vi "Plate Tank 1.vi"() -> ()   [LabVIEW 2019]
uses:
  <vilib>/NI/Current Value Table/Type Defs/Single Tag.ctl
  <vilib>/NI/Current Value Table/Type Defs/Data Types.ctl
  <vilib>/Utility/sysdir.llb/System Directory Type.ctl
  <vilib>/NI/STM/TCP/Read Meta Data (TCP Ref).vi
  <vilib>/NI/STM/TCP/Get Connection Reference (TCP).vi
  <vilib>/NI/AMC/Read Termination Message.vi
  <vilib>/NI/AMC/Create Single Message.vi
  <vilib>/NI/AMC/Update Message Routing Info.vi
  <vilib>/NI/STM/TCP/Read Meta Data (TCP Clst).vi
  <vilib>/NI/AMC/Send Message.vi
  <vilib>/NI/AMC/Globals.vi
  <userlib>/_OpenG.lib/comparison/comparison.llb/I32 Changed__ogtk.vi
  <vilib>/NI/STM/TCP/Write Message (TCP).vi
  <vilib>/NI/AMC/AMC.lvlib
  <vilib>/NI/STM/NI STM.lvlib
  <vilib>/NI/Current Value Table/Current Value Table.lvlib
panel:
  in  "EZ Recipe Button":bool
  out "Loaded Recipe":string
  in  "Load A Recipe":bool
  in  "Save This Recipe":bool
  out "Right Time":dbl format="%.1f"
  out "Left Time":dbl format="%.1f"
  out "Total Amp*min R":dbl format="%.1f"
  out "Total Amp*min L":dbl format="%.1f"
  in  "MO":string
  in  "Reverse Current Multiplier":dbl=3.0 min=0.1 max=100.0 step=0.01 format="%.2g"
  in  "Rectifer Settings":i32(listbox)
  in  "BasT1_P Last Hr":bool
  in  "BasT1_Level Last Hr":bool
  out "Boolean 5":bool
  out "SumpBottom":bool
  out "Process 1 Supply":bool
  out "Sump Return":bool
  out "Boolean 2":bool
  out "SG":dbl format="%.3g"
  out "Return to sump 4":bool
  in  "Rectifer Data":enum32{"Standard", "Eng"}(tab)
  out "Current Step":i32
  out "Left Anode Actual Current":dbl(knob) scale=0.0..150.0
  out "Right Anode Actual Current":dbl(knob) scale=0.0..150.0
  out "Left Anode Amp-min":dbl(slide) scale=0.0..254.0
  out "Right Anode Amp-min":dbl(slide) scale=0.0..135.0
  out "Output Voltage":cluster{dbl, dbl}(graph)
  in  "Tab Control 2":enum32{"Standard", "ENG"}(tab)
  out "Supply Flow":dbl(knob) scale=0.0..65.0
  out "Plating Cell Liquid Level":dbl(slide) scale=0.0..75.0
  out "Cell Temperature":dbl(slide) scale=0.0..60.0
  in  "Cell T Last Hr":bool
  out "Suck Pump":bool
  out "Suck Pump Flow":dbl format="%#_4g"
  out "SuckPipe":bool
  out "SuckPipe 3":bool
  out "Drain Tee Top":bool
  out "Return to sump 2":bool
  out "Return to sump 3":bool
  out "Flow Controller":dbl(knob) scale=0.0..100.0
  in  "Tab Control":enum32{"Main Pump", "Suck Pump"}(tab)
  out "Amps":dbl format="%#.2g"
  out "Volts":dbl format="%#.1f"
  out "VFD T":dbl format="%#.2g"
  out "RPM":dbl format="%#.0f"
  out "Fault Code":dbl format="%#.2g"
  out "Freq":dbl format="%#.2g"
  out "SP1 Amps":dbl caption="Amps" format="%#.2g"
  out "SP1 Volts":dbl caption="Volts" format="%#.1g"
  out "SP1 RPM":dbl caption="RPM" format="%#.2g"
  out "SP1 VFD T":dbl caption="VFD T" format="%#.2g"
  out "SP1 Fault Code":dbl caption="Fault Code" format="%#.2g"
  out "SP1 Freq":dbl caption="Freq" format="%#.2g"
  out "Flow 1":dbl format="%#_4g"
  out "Flow 2":dbl format="%#_4g"
  out "Flow 3":dbl format="%#_4g"
  out "Flow 4":dbl format="%#_4g"
  out "Return to sump":bool
  out "E Stop":bool
  out "Run Enabled?":bool
  in  "Full Drain Plating Cell":bool
  out "Rack Motion":bool
  out "Right Eductor Motion":bool
  out "Left Eductor Motion":bool
  out "Right Output On":bool
  in  "Enable Rack Motion":bool
  in  "Rack RPM":dbl(knob)=1.0 min=1.0 max=11.0 step=0.03 scale=0.0..11.0
  out "Left Output On":bool
  in  "Start Cycle":bool
  in  "Cancel Cycle":bool
  out "SuckPipe 2":bool
  out "Main Pump":bool
  in  "Enable Eductor Motion":bool
  in  "Eductor RPM":dbl(knob)=1.0 min=1.0 max=11.0 step=0.05 scale=0.0..11.0
  in  "Supply Pressure (kPa)":dbl(knob)=50.0 min=50.0 max=200.0 step=5.0 scale=50.0..200.0
  in  "Total Inflow (L/min)":dbl(knob)=40.0 min=25.0 max=50.0 step=0.5 scale=25.0..50.0
  in  "Suck Pump fraction of inflow":dbl(knob)=5.0 min=5.0 max=90.0 step=1.0 scale=0.0..90.0
  out "Sump Level":dbl(slide) scale=0.0..1000.0
  out "Supply Pressure":dbl(knob) scale=0.0..200.0
  in  "Enable Suck Pump":bool
  in  "Enable Plating Cell":bool
  in  "Machine":bool
  in  "Basement 4":bool
  in  "Dryer":bool
  in  "Rinse 4":bool
  in  "Rinse 3":bool
  in  "Rinse 2":bool
  in  "Basement 3":bool
  in  "Basement 2":bool
  in  "Basement 1":bool
  in  "Plater 6":bool
  in  "Plater 5":bool
  in  "Plater 4":bool
  in  "Plater 3":bool
  in  "Plater 2":bool
  in  "Plater 1":bool
  in  "Predip":bool
  in  "Rinse 1":bool
  in  "Cleaner":bool
  in  "Etch":bool
  out "status":string
  out "Boolean 4":bool
  # "Module Selection"
  # "Rectifier Settings"
  # "Fluid Flow Control"
  # "(mins)"
  # "Rectifier Control"
  # "Rectifier Output"
  # "Motion starts when rectifiers cycle"
  # "Note: RPM settings shared with tank 2"
  # "kPa"
  # "@"
  # "Output"
  # "cm"
  # "°C"
  # "L/min"
  # "cm"
  # "L/min"
  # "L/min"
  # "L/min"
  # "L/min"
  # "L/min"
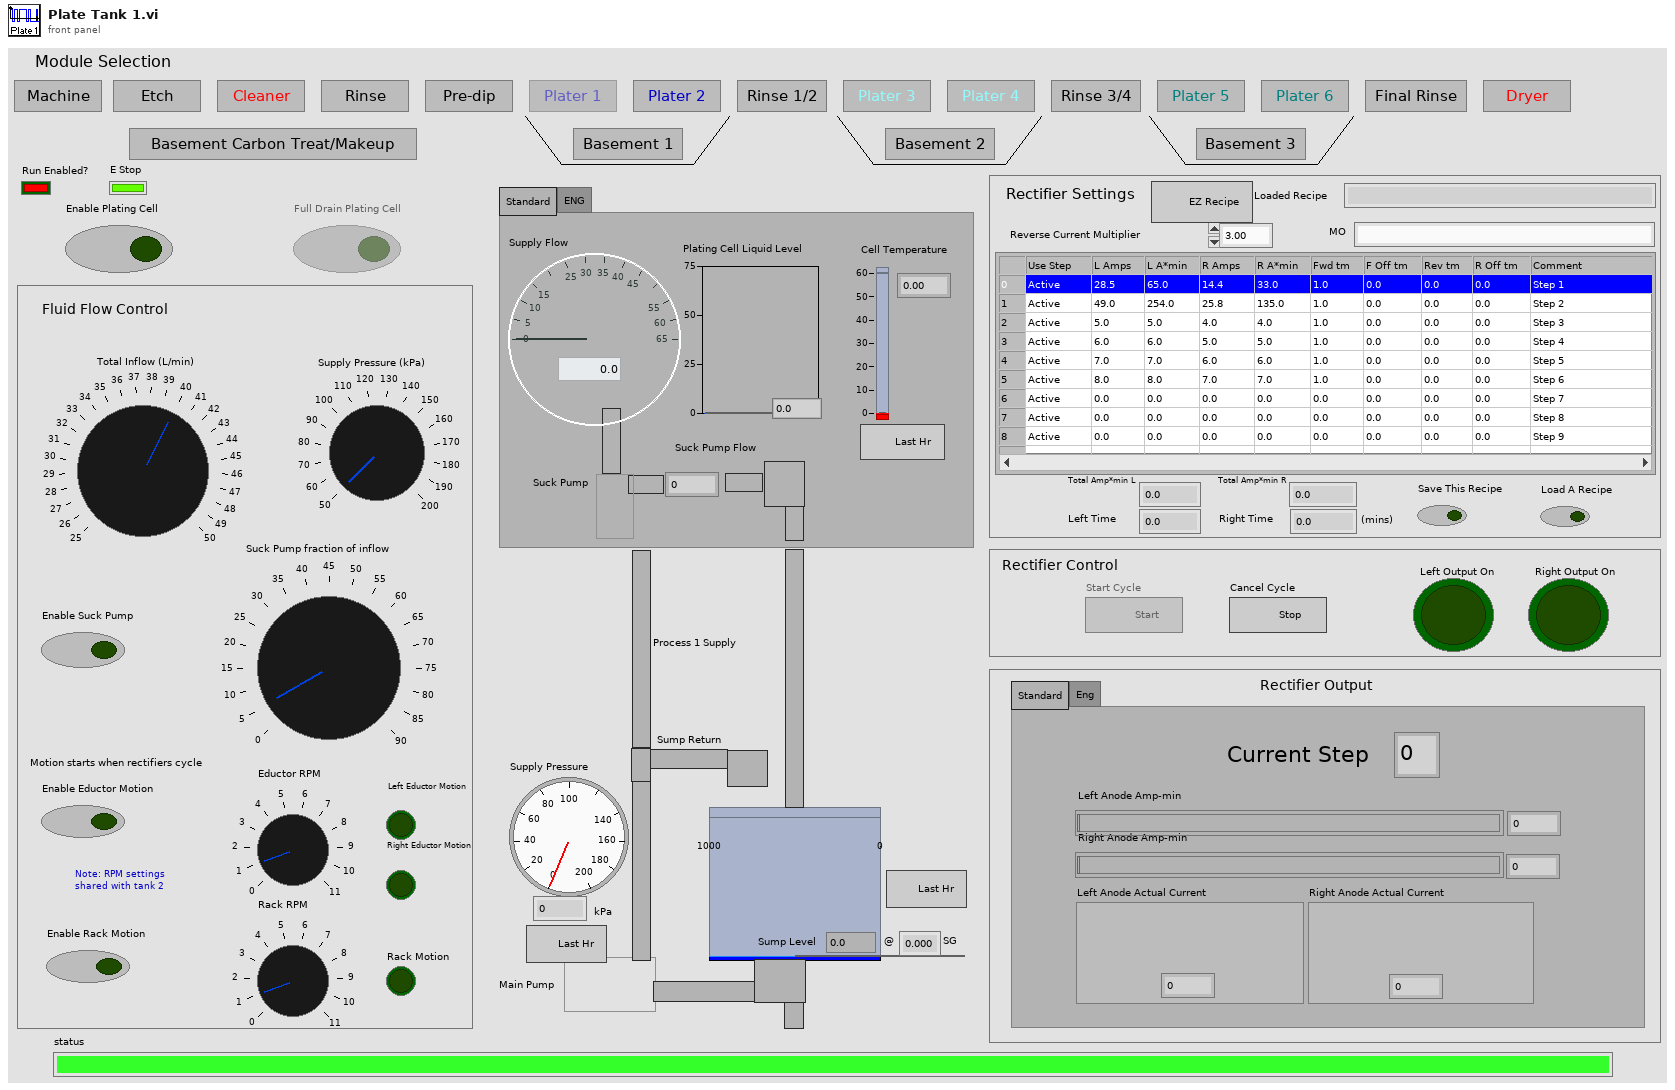
[diagram p1: front panel]
types:
  T1 = typedef "Current Value Table.lvlib/Single Tag.ctl" = cluster{"Data Type":T2, "Name":string, "Value":string, "Description":string}
  T2 = typedef "Current Value Table.lvlib/Data Types.ctl" = enum16{"Double", "Single", "I64", "I32", "I16", "I8", "U64", "U32", "U16", "U8", "String", "Boolean", "Array of U8", "Array of U16", "Array of U32", "Array of U64", "Array of I64", "Array of I32", "Array of I16", "Array of I8", "Array of Double", "Array of Single", "Array of Boolean", "Array of String"}
  T3 = typedef "NI STM.lvlib/TCP Connection Info.ctl" = cluster{"connection ID":refnum<k5>, "meta data":T4[]}
  T4 = typedef "NI STM.lvlib/MetaDataElement.ctl" = string
  T5 = typedef "AMC.lvlib/Message Queue.ctl" = refnum<queue>
  T6 = enum8{"Enabled", "Disabled", "Disabled and Grayed Out"}
  T7 = typedef "System Directory Type.ctl" = i32
  T8 = cluster{"Shift":bool, "Ctrl":bool, "Alt":bool, "Cmd":bool, "Opt":bool}
  T9 = typedef "LVPoint32TypeDef.ctl" = cluster{"Horizontal":i32, "Vertical":i32}
  T10 = typedef "LVRowAndColumnTypeDef.ctl" = cluster{"Row":i32, "Column":i32}
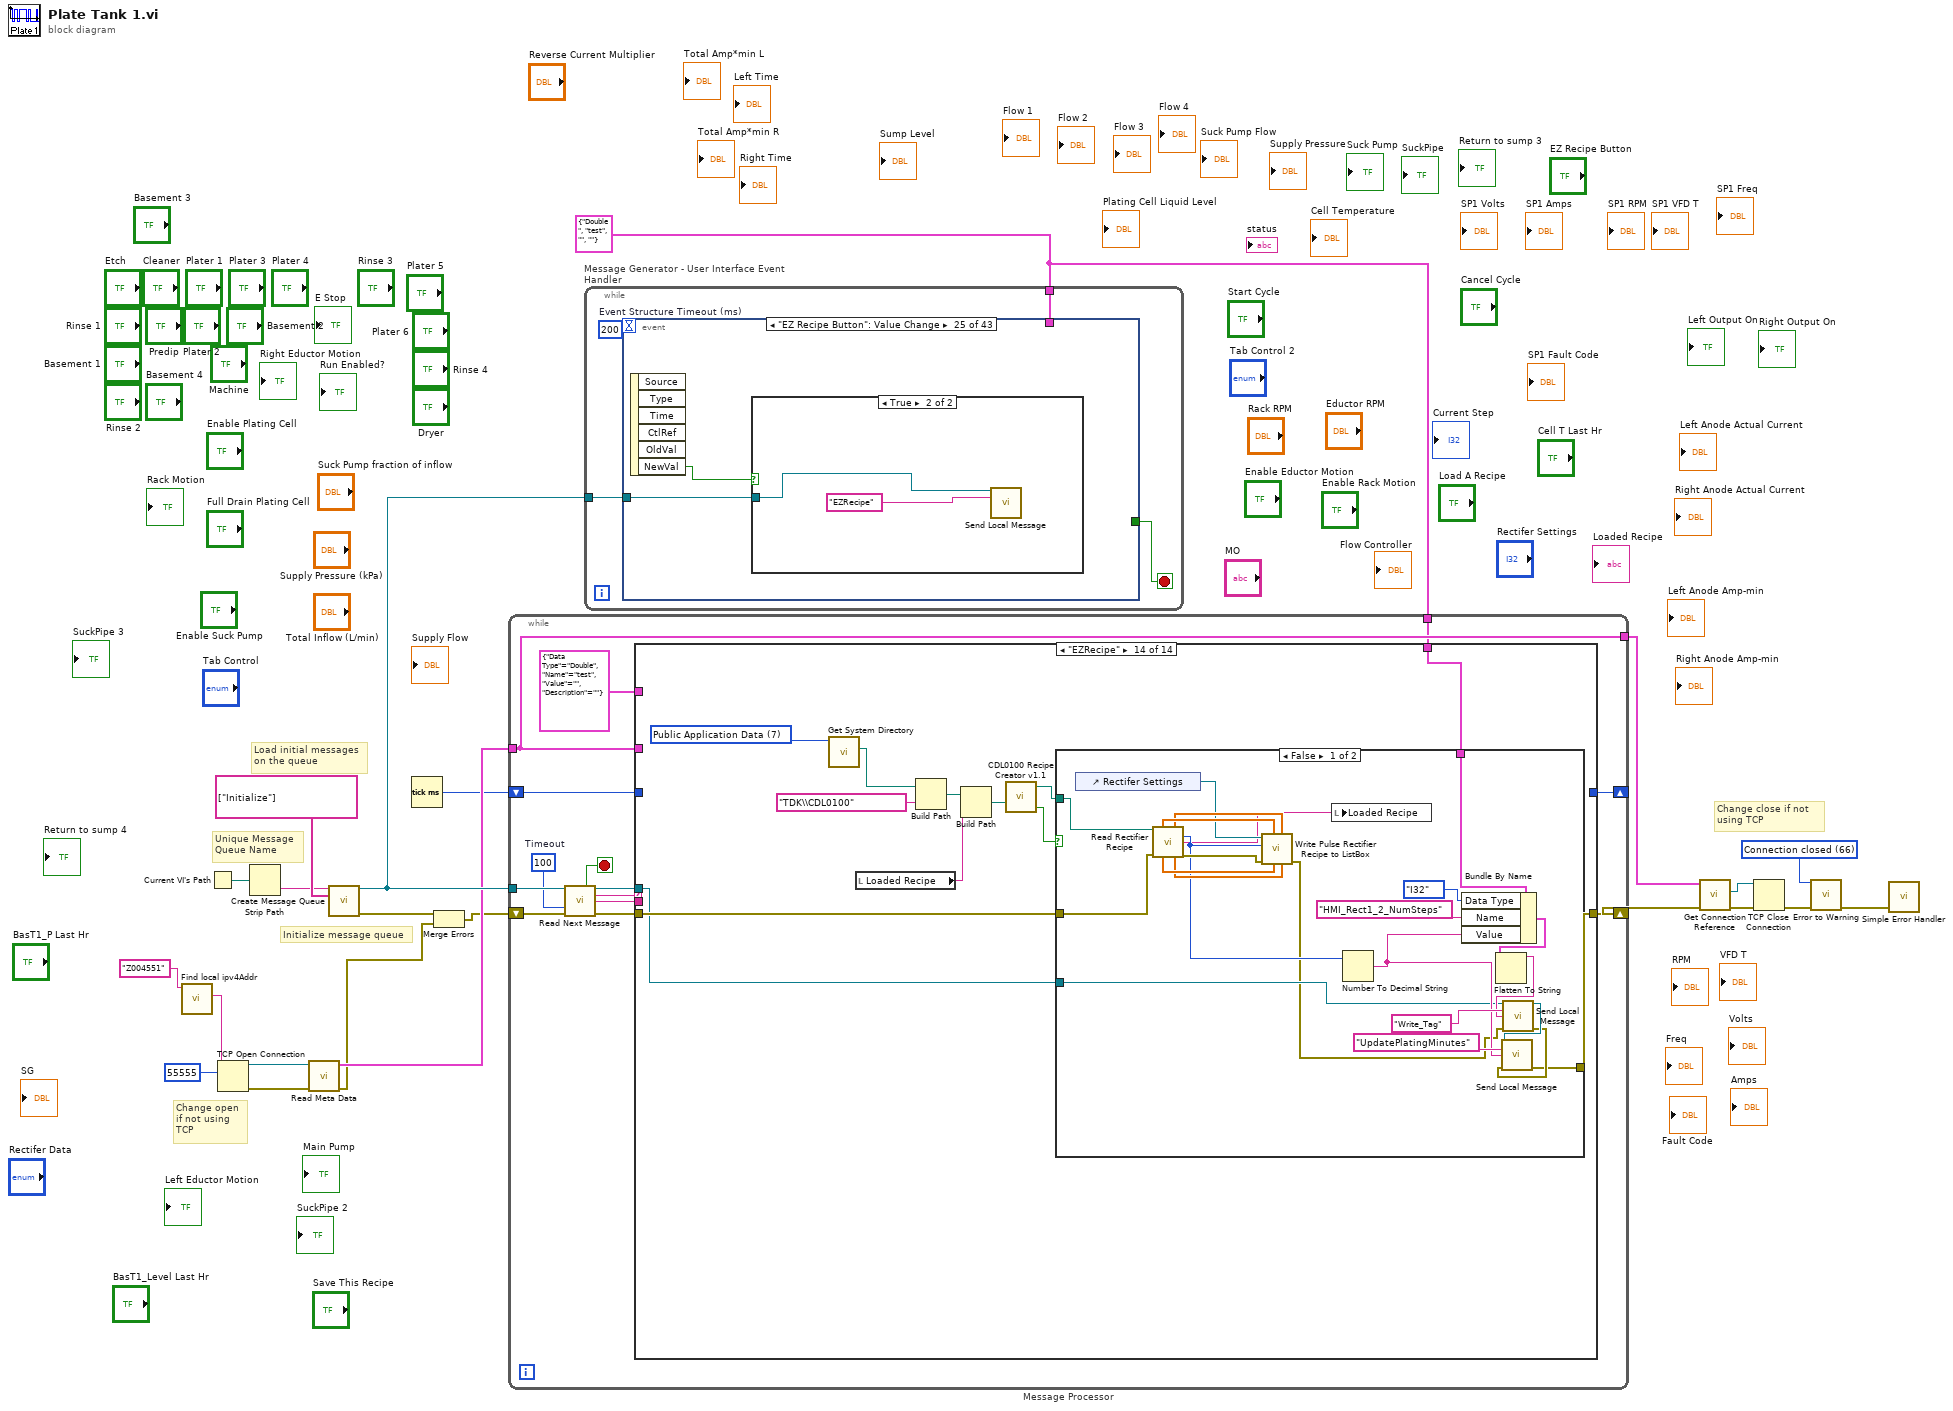
[diagram p0: block diagram]
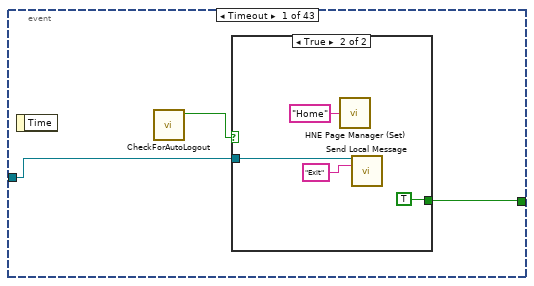
[diagram p2: hidden frame]
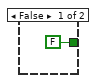
[diagram p3: hidden frame]
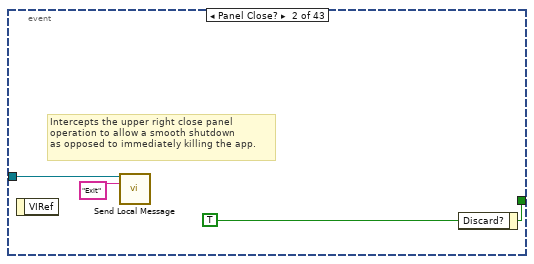
[diagram p4: hidden frame]
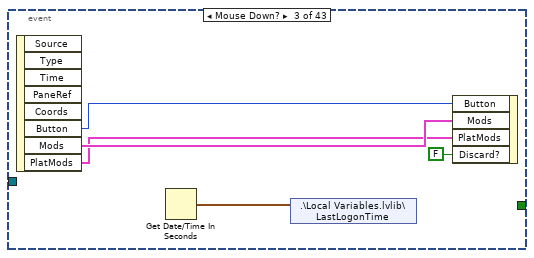
[diagram p5: hidden frame]
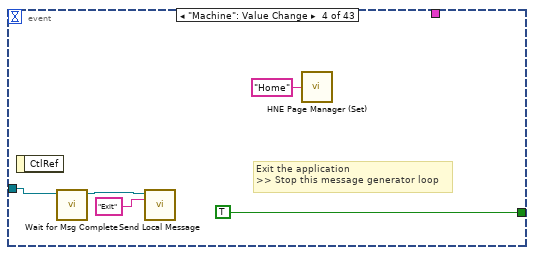
[diagram p6: hidden frame]
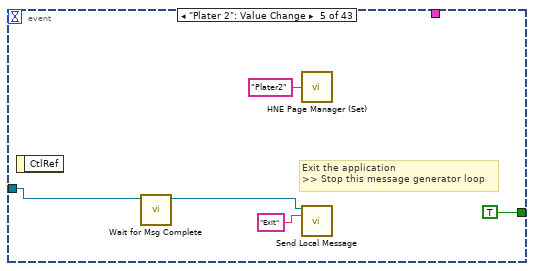
[diagram p7: hidden frame]
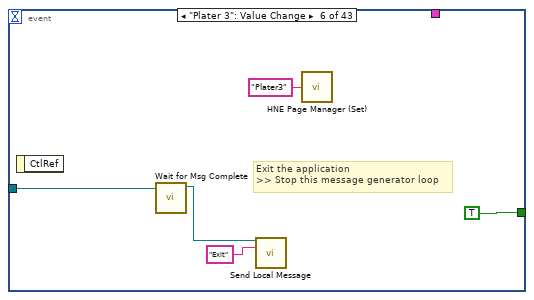
[diagram p8: hidden frame]
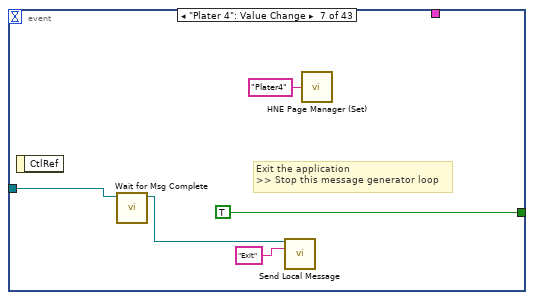
[diagram p9: hidden frame]
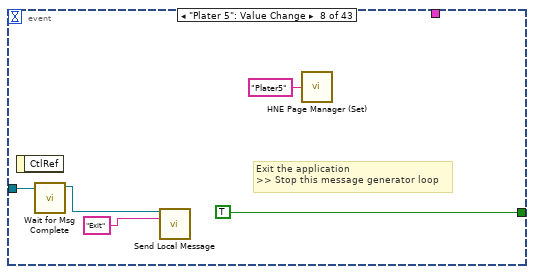
[diagram p10: hidden frame]
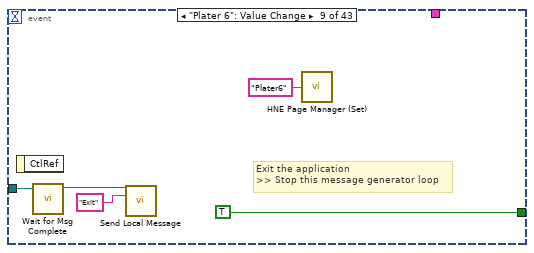
[diagram p11: hidden frame]
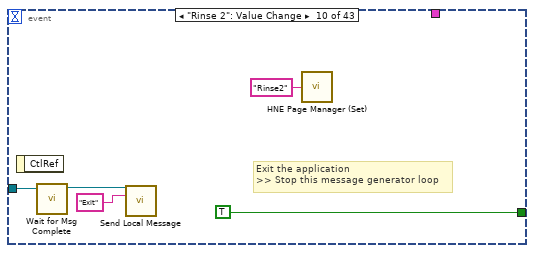
[diagram p12: hidden frame]
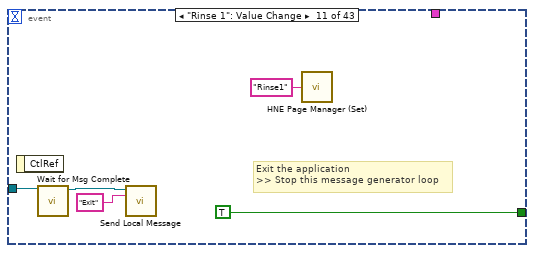
[diagram p13: hidden frame]
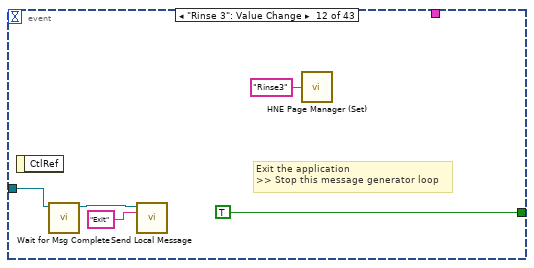
[diagram p14: hidden frame]
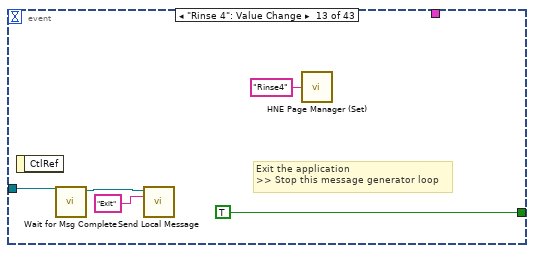
[diagram p15: hidden frame]
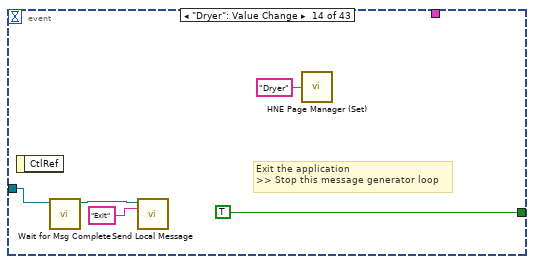
[diagram p16: hidden frame]
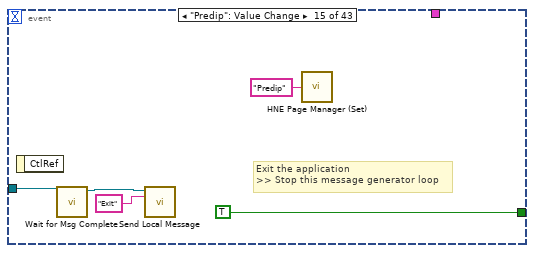
[diagram p17: hidden frame]
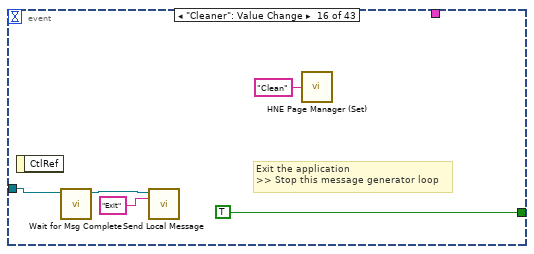
[diagram p18: hidden frame]
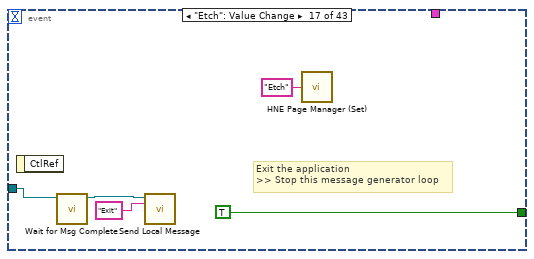
[diagram p19: hidden frame]
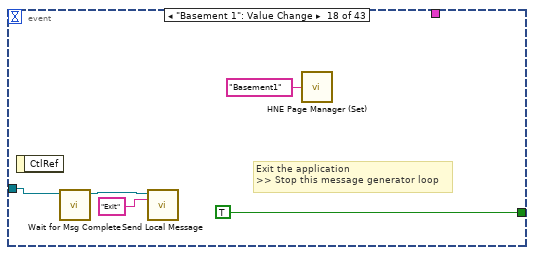
[diagram p20: hidden frame]
diagram:
  w1 = T1 {"Data Type"=enum."Double", "Name"="test", "Value"="", "Description"=""} ("Tag")
  w13 = 66 items=["No Error", "Argument Error", "Memory Full", "Out of Zone", "End of File", "File Already Open", "Generic File IO Error", "File Not Found", "File Permission Error", "Disk Full", "Duplicate Path", "Too Many Files Open", "Not Enabled", "Resource File Not Found", "Cannot Add Resource", "Resource Not Found", "Image Not Found", "Image Memory Error", "Pen Does Not Exist", "Config Bad Type", "Config Token Not Found", "Config Parse Error", "Config Memory Error", "Bad External Code Format", "Bad External Code Offset", "External Code Not Present", "Null Window", "Destroy Window Mixup", "Null Menu", "Print Aborted", "Bad Print Record", "Print Driver Error", "Windows Error During Print", "Memory Error During Print", "Print Dialog Error", "Generic Print Error", "Invalid Device Refnum", "Device Not Found", "Device Parameter Error", "Device Unit Error", "Can't Open Device", "Device Call Aborted", "Generic Error", "Cancelled By User", "Object ID Too Low", "Object ID Too High", "Object Not In Heap", "Unknown Heap", "Bad DefProc ID", "DefProc Not In Table", "Message Out Of Range", "Null Method", "Unknown Message", "Manager Call Not Supported", "Bad address", "Connection In progress", "Connection timed out", "Connection is already in progress", "Network attribute not supported", "Network error", "Address in use", "System out of memory", "Connection aborted", "Connection refused", "Connection is not connected", "Connection is already connected", "Connection closed", "Initialize error (interapplication manager)", "Bad occurrence", "Wait on unbound occurrence handler", "Occurrence queue overflow", "Bad path", "Semaphore not signaled", "Unrecognized type (interapplication manager)"] ("1st Error to Convert")
  # "Change close if not using TCP"
  # "Change open if not using TCP"
  # "Initialize message queue"
  # "Unique Message\nQueue Name"
  # "Load initial messages\non the queue"
  n1 = call "Find local ipv4Addr.vi"("MachineToFind"="Z004551" ("Target IP Address")) -> ("name"=w5:string)  [unwired: 9 in, 1 out]
  n2 = Current VI's Path() -> (path=w19:path)
  n3 = TCP Open Connection(address=w5, remote port or service name=u16 55555 ("remote port")) -> (connection ID=w17:refnum<k5>, error out=w16:errorcluster)  [unwired: 1 in, 2 out]
  n4 = Strip Path(path=w19) -> (name=w21:string)  [unwired: 1 out]
  n5 = call-poly <vilib>:"Read Meta Data.vi"("error in"=w16, "connection ID"=w17) -> ("error out"=w3:errorcluster, "connection info out"=w15:T3)  [unwired: 7 in, 1 out]
  n6 = call <vilib>:"Create Message Queue.vi"("message queue name"=w21, "initial message names"=string[] ["Initialize"]) -> ("message queue out"=w20:T5, "error out"=w4:errorcluster)  [unwired: 12 in]
  n7 = Tick Count (ms)() -> (millisecond timer value=w7:u32)
  n8 = Merge Errors(w4, w3) -> (w2:errorcluster)
  n9 = while "Message Processor" {
    shift-left: w2 -> [w32]
    shift-right: [w36] -> w8
    tunnel: w20 -> [w33]
    tunnel: w15 -> [w27]
    tunnel: [w27] -> w9
    shift-right: [w24] -> _
    shift-left: w7 -> [w25]
    tunnel: w1 -> [w23]
    stop <- w35 stop-if-true
    w28 = 100  # Timeout
    n10 = call <vilib>:"Read Next Message.vi"("message queue in"=w33, "timeout (1 ms)"=w28, "error in"=w32) -> ("exit process?"=w35:bool, "message queue out"=w34:T5, "message name"=w30:string, "message value"=w29:string, "error out"=w31:errorcluster)  [unwired: 5 in, 3 out]
    n11 = case shown="\"EZRecipe\"" w30 {
      selector: w30 -> [_ _ w129 _ _ _ _ _ _ _ _ _ _ _]
      tunnel: w34 -> [_ _ _ _ _ w134 w277 _ _ _ w299 _ w325 w353]
      tunnel: w31 -> [w37 w49 w130 w131 w133 w136 w278 w280 w284 w287 w297 w316 w323 w355]
      tunnel: [w37 w49 w130 errorcluster {"status"=FALSE, "code"=0, "source"=""} ("error out") w133 w136 w276 w280 w283 w287 w290 w306 w326 w352] -> w36
      tunnel: w29 -> [_ _ _ _ _ _ _ _ w282 w289 w301 _ _ _]
      tunnel: w27 -> [_ _ _ _ _ _ _ _ w285 _ _ _ _ _]
      tunnel: T1 {"Data Type"=enum."Double", "Name"="test", "Value"="", "Description"=""} ("Tag") -> [_ _ _ _ _ _ _ _ _ _ _ _ _ _]
      tunnel: w25 -> [_ w44 _ _ _ w135 _ _ w281 w288 w302 w317 _ _]
      tunnel: [_ w45 _ _ _ w135 _ _ w281 w288 w302 w317 _ _] -> w24
      tunnel: w23 -> [_ _ _ _ _ _ _ _ _ _ _ _ w324 w354]
      frame "---------- Framework Operations ----------" {
        # "Dummy case to add a seperator in the Case Structure menu"
      }
      frame "", "Idle" {
        n12 = stacked-sequence {
          frame #0 {
            n13 = shared-variable-read(refnum<k21> "ni.var.psp://z004551/CDL0100 ReadTags/Tnk1_Can_Plate" ("shared variable refnum in"), FALSE) -> (w64:bool)  [unwired: 1 in, 3 out]
            n14 = shared-variable-read(refnum<k21> "ni.var.psp://z004551/CDL0100 ReadWriteTags/HMI_Tank1_Drain" ("shared variable refnum in"), FALSE) -> (w53:bool)  [unwired: 1 in, 3 out]
            n15 = control-ref of="Start Cycle"() -> (w66:refnum<vi>)
            n16 = shared-variable-read(refnum<k21> "ni.var.psp://z004551/CDL0100 ReadWriteTags/HMI_Enable_BTnk1_Pump" ("shared variable refnum in"), FALSE) -> (w50:bool)  [unwired: 1 in, 3 out]
            n17 = shared-variable-read(refnum<k21> "ni.var.psp://z004551/CDL0100 ReadWriteTags/HMI_Tank1_Enable" ("shared variable refnum in"), FALSE) -> (w59:bool)  [unwired: 1 in, 3 out]
            n18 = case shown="False" w64 {
              tunnel: [T6."Disabled and Grayed Out" ("Disabled") T6."Enabled" ("Disabled")] -> w65
              frame False {
              }
              frame True {
              }
            }
            n19 = Or(x=w59, y=w50) -> (x .or. y?=w58:bool)
            n20 = case shown="True" w53 {
              tunnel: [T6."Enabled" ("Disabled") T6."Disabled and Grayed Out" ("Disabled")] -> w52
              frame False {
              }
              frame True {
              }
            }
            n21 = case shown="True" w58 {
              tunnel: [T6."Enabled" ("Disabled") T6."Disabled and Grayed Out" ("Disabled")] -> w57
              frame False {
              }
              frame True {
              }
            }
            n22 = control-ref of="Full Drain Plating Cell"() -> (w56:refnum<vi>)
            n23 = control-ref of="Enable Plating Cell"() -> (w51:refnum<vi>)
            n24 = property class="Bool (strict)"(reference=w66, "DisabledEnum"=w65) -> ()  [unwired: 1 in, 2 out]
            n25 = property class="Bool (strict)"(reference=w51, "DisabledEnum"=w52) -> ()  [unwired: 1 in, 2 out]
            n26 = property class="Bool (strict)"(reference=w56, "DisabledEnum"=w57) -> ()  [unwired: 1 in, 2 out]
          }
          frame #1 {
            n27 = shared-variable-read(refnum<k21> "ni.var.psp://z004551/CDL0100 ReadTags/IO_Bas_Tnk1_3Way_At_Recirc" ("shared variable refnum in"), FALSE) -> (w78:bool)  [unwired: 1 in, 3 out]
            n28 = shared-variable-read(refnum<k21> "ni.var.psp://z004551/CDL0100 ReadTags/IO_Bas_Tnk1_3Way_At_Open" ("shared variable refnum in"), FALSE) -> (w79:bool)  [unwired: 1 in, 3 out]
            n29 = shared-variable-read(refnum<k21> "ni.var.psp://z004551/CDL0100 ReadTags/IO_Bas_Tnk1_3Way_At_Closed" ("shared variable refnum in"), FALSE) -> (w82:bool)  [unwired: 1 in, 3 out]
            n30 = Or(x=w79, y=w78) -> (x .or. y?=w76:bool)
            "Sump Return" <- w76
            "Boolean 2" <- w76
            n31 = Or(x=w82, y=w79) -> (x .or. y?=w77:bool)
            "Return to sump" <- w77
            "Drain Tee Top" <- w77
            "Return to sump 2" <- w77
            "Process 1 Supply" <- w77
            n32 = Or(x=w77, y=w76) -> (x .or. y?=→"Boolean 5":bool)
          }
          frame #2 {
            n33 = shared-variable-read(refnum<k21> "ni.var.psp://z004551/CDL0100 ReadWriteTags/HMI_Tank1_Drain" ("shared variable refnum in"), FALSE) -> (w87:bool)  [unwired: 1 in, 3 out]
            "Boolean 4" <- w87
            n34 = shared-variable-read(refnum<k21> "ni.var.psp://z004551/CDL0100 ReadWriteTags/HMI_Enable_BTnk1_Pump" ("shared variable refnum in"), FALSE) -> (w88:bool)  [unwired: 1 in, 3 out]
            n35 = Or(x=w88, y=w87) -> (x .or. y?=→"SumpBottom":bool)
          }
          frame #3 {
            n36 = shared-variable-read(refnum<k21> "ni.var.psp://z004551/CDL0100 ReadTags/Rect1_2_CurrRecpStp" ("shared variable refnum in"), 0) -> (w94:i32)  [unwired: 1 in, 3 out]
            n37 = call-poly <userlib>:"Data Changed__ogtk.vi"("I32"=w94) -> ("Changed"=w97:bool)
            n38 = case shown="True" w97 {
              tunnel: w94 -> [_ w99]
              frame False {
              }
              frame True {
                w104 = 0.0 ("Scale.Range:Minimum")
                n39 = shared-variable-read(refnum<k21> "ni.var.psp://z004551/CDL0100 ReadWriteTags/HMI_Rect1_2_NumSteps" ("shared variable refnum in"), 0) -> (w98:i32)  [unwired: 1 in, 3 out]
                n40 = Less?(x=w99, y=w98) -> (x < y?=w112:bool)
                n41 = case shown="False" w112 {
                  tunnel: w99 -> [w116 w117]
                  tunnel: [w115 w117] -> w111
                  frame False {
                    n42 = Decrement(x=w116) -> (x-1=w115:i32)
                  }
                  frame True {
                  }
                }
                n43 = shared-variable-read(refnum<k21> "ni.var.psp://z004551/CDL0100 ReadWriteTags/HMI_Rct2_AMin_SetPnts" ("shared variable refnum in"), dbl[] []) -> (w105:dbl[])  [unwired: 1 in, 3 out]
                n44 = Index Array(array=w105, index=w111) -> (element=w102:dbl)
                n45 = control-ref of="Right Anode Amp-min"() -> (w100:refnum<vi>)
                n46 = shared-variable-read(refnum<k21> "ni.var.psp://z004551/CDL0100 ReadWriteTags/HMI_Rct1_AMin_SetPnts" ("shared variable refnum in"), dbl[] []) -> (w108:dbl[])  [unwired: 1 in, 3 out]
                n47 = Index Array(array=w108, index=w111) -> (element=w103:dbl)
                n48 = control-ref of="Left Anode Amp-min"() -> (w101:refnum<vi>)
                n49 = property class="Slide (strict)"(reference=w101, "Scale.Maximum"=w103, "Scale.Minimum"=w104) -> ()  [unwired: 1 in, 2 out]
                n50 = property class="Slide (strict)"(reference=w100, "Scale.Maximum"=w102, "Scale.Minimum"=w104) -> ()  [unwired: 1 in, 2 out]
              }
            }
          }
        }
        n51 = local read "Left Output On"() -> (w41:bool)
        n52 = local read "Right Output On"() -> (w42:bool)
        n53 = control-ref of="status"() -> (w48:refnum<vi>)
        n54 = Tick Count (ms)() -> (millisecond timer value=w43:u32)
        n55 = Subtract(x=w43, y=w44) -> (x-y=w46:u32)
        n56 = Or(x=w41, y=w42) -> (x .or. y?=w40:bool)
        n57 = call <userlib>:"TAE Format Alarm Ticker.vi"("Alarm Ticker Ref"=w48) -> ()  [unwired: 15 in]
        n58 = Greater?(x=w46, y=u32 500) -> (0:w39:bool)
        n59 = And(x=w40, y=w39) -> (x .and. y?=w38:bool)
        n60 = case shown="True" w38 {
          tunnel: w43 -> [_ w119]
          tunnel: [w118 w119] -> w45
          tunnel: w44 -> [w118 _]
          frame False {
          }
          frame True {
            n61 = shared-variable-read(refnum<k21> "ni.var.psp://z004551/CDL0100 ReadTags/Rect1_ActlVolts" ("shared variable refnum in"), 0.0) -> (w122:dbl)  [unwired: 1 in, 3 out]
            n62 = shared-variable-read(refnum<k21> "ni.var.psp://z004551/CDL0100 ReadTags/Rect2_ActlVolts" ("shared variable refnum in"), 0.0) -> (w121:dbl)  [unwired: 1 in, 3 out]
            n63 = Bundle(w122, w121) -> (→"Output Voltage":cluster{dbl, dbl})  [unwired: 1 in]
          }
        }
      }
      frame "Missing Message Handler", Default {
        # "Call this case if a message is received that is not handled \nby any other case. Typically this is a programming error\nas a result of a typo or unhandled message/missing message handler."
        n64 = Format Into String(format string="DevError: Missing message handler for '%s\" message." ("message"), w129) -> (resulting string=w127:string)  [unwired: 2 in, 1 out]
        n65 = One Button Dialog(message=w127) -> ()  [unwired: 2 out]
      }
      frame "Error" {
        # "General Error Case - this case is called if an error is passed using the error cluster below. Typically most new errors should be handed in each individual case and not passed in the rror cluster. If necessary a custom error handler case should be added and called from other cases."
        n66 = call <vilib>:"Simple Error Handler.vi"("error in (no error)"=w131) -> ()  [unwired: 1 in, 8 out]
      }
      frame "---------- Generic Operations ----------" {
        # "Dummy case to add a seperator in the Case Structure menu"
      }
      frame "Initialize" {
        n67 = stacked-sequence {
          seq-local: [_ w162 _ _ _] -> [_ _ _ w208 w264]
          seq-local: [_ w166 _ _ _] -> [_ _ _ w207 _]
          seq-local: [_ w159 _ _ _] -> [_ _ _ w206 w263]
          seq-local: [_ _ w198 _ _] -> [_ _ _ w205 _]
          seq-local: [_ _ w195 _ _] -> [_ _ _ w204 _]
          seq-local: [_ _ w192 _ _] -> [_ _ _ w203 _]
          seq-local: [_ _ w189 _ _] -> [_ _ _ w202 _]
          seq-local: [w137 _ _ _ _] -> [_ w158 _ w201 w257]
          tunnel: w134 -> [_ _ _ _ w272]
          frame #0 {
            n68 = shared-variable-read(refnum<k21> "ni.var.psp://z004551/CDL0100 ReadWriteTags/HMI_TNK1_SuckPmpFrac_Setpoint" ("shared variable refnum in"), 0.0) -> (w142:dbl)  [unwired: 1 in, 3 out]
            n69 = shared-variable-read(refnum<k21> "ni.var.psp://z004551/CDL0100 ReadWriteTags/HMI_Tnk1_Enable_SuckPump" ("shared variable refnum in"), FALSE) -> (w145:bool)  [unwired: 1 in, 3 out]
            n70 = shared-variable-read(refnum<k21> "ni.var.psp://z004551/CDL0100 ReadWriteTags/HMI_Tnk1_Rack_RPM" ("shared variable refnum in"), 0.0) -> (w156:dbl)  [unwired: 1 in, 3 out]
            n71 = shared-variable-read(refnum<k21> "ni.var.psp://z004551/CDL0100 ReadWriteTags/HMI_Tank1_Rack_Motor_Run" ("shared variable refnum in"), FALSE) -> (w155:bool)  [unwired: 1 in, 3 out]
            n72 = shared-variable-read(refnum<k21> "ni.var.psp://z004551/CDL0100 ReadWriteTags/HMI_TNK1_Flow_Setpoint" ("shared variable refnum in"), 0.0) -> (w154:dbl)  [unwired: 1 in, 3 out]
            n73 = Multiply(x=w142, y=100.0) -> (x*y=w140:dbl)
            n74 = local write "Enable Suck Pump"(w145) -> ()
            n75 = local write "Rack RPM"(w156) -> ()
            n76 = local write "Enable Rack Motion"(w155) -> ()
            n77 = shared-variable-read(refnum<k21> "ni.var.psp://z004551/CDL0100 ReadWriteTags/HMI_Rect1_2_NumSteps" ("shared variable refnum in"), 0) -> (w137:i32)  [unwired: 1 in, 3 out]
            n78 = local write "Total Inflow (L/min)"(w154) -> ()
            n79 = local write "Suck Pump fraction of inflow"(w140) -> ()
          }
          frame #1 {
            n80 = shared-variable-read(refnum<k21> "ni.var.psp://z004551/CDL0100 ReadWriteTags/HMI_Rct1_AMin_SetPnts" ("shared variable refnum in"), dbl[] []) -> (w162:dbl[])  [unwired: 1 in, 3 out]
            n81 = shared-variable-read(refnum<k21> "ni.var.psp://z004551/CDL0100 ReadWriteTags/HMI_Rct2_AFwd_SetPnts" ("shared variable refnum in"), dbl[] []) -> (w166:dbl[])  [unwired: 1 in, 3 out]
            n82 = shared-variable-read(refnum<k21> "ni.var.psp://z004551/CDL0100 ReadWriteTags/HMI_Rct2_AMin_SetPnts" ("shared variable refnum in"), dbl[] []) -> (w159:dbl[])  [unwired: 1 in, 3 out]
            n83 = for {
              N: w158 -> [_]
              tunnel: w159 -> [w185] mode=indexing
              shift-right: [w183] -> w157
              shift-left: 0.0 -> [w184]
              n84 = Add(x=w185, y=w184) -> (x+y=w183:dbl)
            }
            n85 = for {
              N: w158 -> [_]
              tunnel: w162 -> [w188] mode=indexing
              shift-right: [w186] -> w161
              shift-left: 0.0 -> [w187]
              n86 = Add(x=w188, y=w187) -> (x+y=w186:dbl)
            }
            n87 = shared-variable-read(refnum<k21> "ni.var.psp://z004551/CDL0100 ReadWriteTags/HMI_Tank1_Drain" ("shared variable refnum in"), FALSE) -> (w171:bool)  [unwired: 1 in, 3 out]
            n88 = shared-variable-read(refnum<k21> "ni.var.psp://z004551/CDL0100 ReadWriteTags/HMI_Tnk1_Eductor_RPM" ("shared variable refnum in"), 0.0) -> (w179:dbl)  [unwired: 1 in, 3 out]
            n89 = shared-variable-read(refnum<k21> "ni.var.psp://z004551/CDL0100 ReadWriteTags/HMI_Tank1_Eductor_Motors_Run" ("shared variable refnum in"), FALSE) -> (w182:bool)  [unwired: 1 in, 3 out]
            n90 = shared-variable-read(refnum<k21> "ni.var.psp://z004551/CDL0100 ReadWriteTags/HMI_Tank1_Enable" ("shared variable refnum in"), FALSE) -> (w178:bool)  [unwired: 1 in, 3 out]
            n91 = local write "Full Drain Plating Cell"(w171) -> ()
            n92 = local write "Enable Eductor Motion"(w182) -> ()
            n93 = local write "Enable Plating Cell"(w178) -> ()
            n94 = local write "Eductor RPM"(w179) -> ()
            n95 = local write "Total Amp*min R"(w157) -> ()
            n96 = local write "Total Amp*min L"(w161) -> ()
          }
          frame #2 {
            n97 = shared-variable-read(refnum<k21> "ni.var.psp://z004551/CDL0100 ReadWriteTags/HMI_Rct1_FwdOffTm_SetPnts" ("shared variable refnum in"), dbl[] []) -> (w195:dbl[])  [unwired: 1 in, 3 out]
            n98 = shared-variable-read(refnum<k21> "ni.var.psp://z004551/CDL0100 ReadWriteTags/HMI_Rct1_FwdTm_SetPnts" ("shared variable refnum in"), dbl[] []) -> (w198:dbl[])  [unwired: 1 in, 3 out]
            n99 = shared-variable-read(refnum<k21> "ni.var.psp://z004551/CDL0100 ReadWriteTags/HMI_Rct1_BwdTm_SetPnts" ("shared variable refnum in"), dbl[] []) -> (w192:dbl[])  [unwired: 1 in, 3 out]
            n100 = shared-variable-read(refnum<k21> "ni.var.psp://z004551/CDL0100 ReadWriteTags/HMI_Rct1_BwdOffTm_SetPnts" ("shared variable refnum in"), dbl[] []) -> (w189:dbl[])  [unwired: 1 in, 3 out]
          }
          frame #3 {
            n101 = control-ref of="Rectifer Settings"() -> (w216:refnum<vi>)
            n102 = shared-variable-read(refnum<k21> "ni.var.psp://z004551/CDL0100 ReadWriteTags/HMI_Rct1_AFwd_SetPnts" ("shared variable refnum in"), dbl[] []) -> (w210:dbl[])  [unwired: 1 in, 3 out]
            n103 = for {
              N: 10 -> [_]
              tunnel: [w255] -> w214 mode=indexing
              tunnel: [w253] -> w209 mode=indexing
              tunnel: w210 -> [w251] mode=indexing
              tunnel: w208 -> [w248] mode=indexing
              tunnel: w207 -> [w245] mode=indexing
              tunnel: w206 -> [w242] mode=indexing
              tunnel: w205 -> [w239] mode=indexing
              tunnel: w204 -> [w236] mode=indexing
              tunnel: w203 -> [w233] mode=indexing
              tunnel: w202 -> [w230] mode=indexing
              i -> [w227]
              n104 = Number To Fractional String(number=w239, precision (6)=i16 1) -> (F-format string=w238:string)  [unwired: 2 in]
              n105 = Number To Fractional String(number=w242, precision (6)=i16 1) -> (F-format string=w241:string)  [unwired: 2 in]
              n106 = Number To Fractional String(number=w248, precision (6)=i16 1) -> (F-format string=w247:string)  [unwired: 2 in]
              n107 = Number To Fractional String(number=w245, precision (6)=i16 1) -> (F-format string=w244:string)  [unwired: 2 in]
              n108 = Number To Fractional String(number=w251, precision (6)=i16 1) -> (F-format string=w250:string)  [unwired: 2 in]
              n109 = Number To Fractional String(number=w236, precision (6)=i16 1) -> (F-format string=w235:string)  [unwired: 2 in]
              n110 = Number To Fractional String(number=w233, precision (6)=i16 1) -> (F-format string=w232:string)  [unwired: 2 in]
              n111 = Increment(x=w227) -> (x+1=w226:i32)
              n112 = Number To Decimal String(number=w227) -> (decimal integer string=w255:string)  [unwired: 1 in]
              n113 = Number To Fractional String(number=w230, precision (6)=i16 1) -> (F-format string=w229:string)  [unwired: 2 in]
              n114 = call "Build Text"("d"=w226) -> ("Result"=w228:string)  [unwired: 13 in, 1 out]
              n115 = Build Array("Active", w250, w247, w244, w241, w238, w235, w232, w229, w228) -> (w253:string[])
            }
            n116 = shared-variable-read(refnum<k21> "ni.var.psp://z004551/CDL0100 ReadWriteTags/HMI_BAS_TNK1_P_Setpoint" ("shared variable refnum in"), 0.0) -> (w223:dbl)  [unwired: 1 in, 3 out]
            n117 = local write "Supply Pressure (kPa)"(w223) -> ()
            n118 = Subtract(x=10, y=w201) -> (x-y=w219:i32)
            n119 = Initialize Array(38, w201) -> (w218:i32[])
            n120 = Initialize Array(37, w219) -> (w217:i32[])
            n121 = Build Array (concatenate)(w218, w217) -> (w215:i32[])
            n122 = property class="MCListbox (strict)"(reference=w216, "ItemSyms"=w215, "RowHdrs[]"=w214, "ItemNames"=w209) -> ()  [unwired: 1 in, 2 out]
          }
          frame #4 {
            w260 = 0.0 ("Scale.Range:Minimum")
            n123 = Number To Decimal String(number=w257) -> (decimal integer string=w270:string)  [unwired: 1 in]
            n124 = shared-variable ".\\Local Variables.lvlib\\PT1_MO"() -> (w269:string)  [unwired: 1 in, 1 out]
            n125 = shared-variable-read(refnum<k21> "ni.var.psp://z004551/CDL0100 ReadTags/Rect1_2_CurrRecpStp" ("shared variable refnum in"), 0) -> (w256:i32)  [unwired: 1 in, 3 out]
            n126 = Less?(x=w256, y=w257) -> (x < y?=w266:bool)
            n127 = local write "MO"(w269) -> ()
            n128 = case shown="False" w266 {
              tunnel: w256 -> [w274 w275]
              tunnel: [w273 w275] -> w265
              frame False {
                n129 = Decrement(x=w274) -> (x-1=w273:i32)
              }
              frame True {
              }
            }
            n130 = call <vilib>:"Send Local Message.vi"("message queue in"=w272, "message name"="UpdatePlatingMinutes", "message value"=w270) -> ()  [unwired: 10 in, 3 out]
            n131 = Index Array(array=w263, index=w265) -> (element=w259:dbl)
            n132 = Index Array(array=w264, index=w265) -> (element=w261:dbl)
            n133 = control-ref of="Left Anode Amp-min"() -> (w262:refnum<vi>)
            n134 = control-ref of="Right Anode Amp-min"() -> (w258:refnum<vi>)
            n135 = property class="Slide (strict)"(reference=w262, "Scale.Maximum"=w261, "Scale.Minimum"=w260) -> ()  [unwired: 1 in, 2 out]
            n136 = property class="Slide (strict)"(reference=w258, "Scale.Maximum"=w259, "Scale.Minimum"=w260) -> ()  [unwired: 1 in, 2 out]
          }
        }
      }
      frame "Exit" {
        # "Destroy message queue >> this will halt the UI event handler loop"
        # "Stop the VI\n>> Perform any cleanup tasks in this message case.\n>> Clear display before closing."
        n137 = call <vilib>:"Destroy Message Queue.vi"("message queue in"=w277, "error in"=w278) -> ("error out"=w276:errorcluster)  [unwired: 11 in, 2 out]
        n138 = local write "status"("" ("Status")) -> ()
      }
      frame "---------- Application Operations ----------" {
        # "Dummy case to add a seperator in the Case Structure menu"
      }
      frame "Write_Tag" {
        n139 = call-poly <vilib>:"Write Message.vi"("error in"=w284, "data"=w282, "name"="WriteTag", "connection info in"=w285) -> ("error out"=w283:errorcluster)  [unwired: 6 in, 1 out]
      }
      frame "DisplayLastHr" {
        n140 = call "Trace Variable 1 hour Popup.vi"("Tag"=w289) -> ()  [unwired: 11 in]
      }
      frame "UpdatePlatingMinutes" {
        n141 = Decimal String To Number(string=w301) -> (number=w295:i32)  [unwired: 2 in, 1 out]
        n142 = control-ref of="Rectifer Settings"() -> (w300:refnum<vi>)
        n143 = local read "Reverse Current Multiplier"() -> (w298:dbl)
        n144 = call "Assemble Rectifier Setting Changes for PLC.vi"("Num Steps"=w295, "Rect Number"=1, "error In"=w297, "Reverse Current Multiplier"=w298, "message queue in"=w299, "MulticolumnListbox in"=w300) -> ("Right Anode Mins"=w291:dbl, "Left Anode Mins"=w292:dbl, "Right AmpMin"=w293:dbl, "Left AmpMin"=w294:dbl, "error out"=w290:errorcluster)  [unwired: 1 in]
        n145 = local write "Total Amp*min L"(w294) -> ()
        n146 = local write "Total Amp*min R"(w293) -> ()
        n147 = local write "Left Time"(w292) -> ()
        n148 = local write "Right Time"(w291) -> ()
      }
      frame "Save_Recipe" {
        n149 = control-ref of="Rectifer Settings"() -> (w315:refnum<vi>)
        n150 = local read "Reverse Current Multiplier"() -> (w305:dbl)
        n151 = call "Convert RectifierListData to Arrays.vi"("MulticolumnListbox in"=w315, "error in (no error)"=w316) -> ("Left Amps"=w314:dbl[], "Right Amps"=w313:dbl[], "Left AmpMins"=w312:dbl[], "Right Amp Min"=w310:dbl[], "error out"=w311:errorcluster)  [unwired: 5 in, 4 out]
        n152 = shared-variable-read(refnum<k21> "ni.var.psp://z004551/CDL0100 ReadWriteTags/HMI_Rect1_2_NumSteps" ("shared variable refnum in"), 0) -> (w307:i32)  [unwired: 1 in, 3 out]
        n153 = call "Save Rectifier Recipe.vi"("Rev Mult"=w305, "Right AmpMins"=w310, "Left AmpMins"=w312, "error in"=w311, "Number Steps"=w307, "Right Amps"=w313, "Left Amps"=w314) -> ("error out"=w306:errorcluster, "name"=w303:string, "cancelled"=w304:bool)  [unwired: 2 in]
        n154 = case shown="False" w304 {
          tunnel: w303 -> [w318 _]
          frame False {
            n155 = local write "Loaded Recipe"(w318) -> ()
          }
          frame True {
          }
        }
      }
      frame "Load_A_Recipe" {
        n156 = call "BrowseRecipe.vi"("error in (no error)"=w323) -> ("error out"=w321:errorcluster, "cancelled"=w322:bool, "selected path"=w320:path)  [unwired: 8 in]
        n157 = control-ref of="Rectifer Settings"() -> (w319:refnum<vi>)
        n158 = case shown="False" w322 {
          tunnel: w321 -> [w332 w351]
          tunnel: [w329 w351] -> w326
          tunnel: w325 -> [w342 _]
          tunnel: w324 -> [w341 _]
          tunnel: w320 -> [w331 _]
          tunnel: w319 -> [w330 _]
          frame False {
            n159 = call "Read Rectifier Recipe.vi"("selected path"=w331, "error in"=w332) -> ("Left Amps"=w338:dbl[], "Left AmpMins"=w337:dbl[], "Num Steps"=w336:i32, "name"=w328:string, "Rev Mult"=w327:dbl, "Right Amps"=w335:dbl[], "Right AmpMins"=w334:dbl[], "error out"=w333:errorcluster)  [unwired: 5 in, 1 out]
            n160 = local write "Loaded Recipe"(w328) -> ()
            n161 = call "Write Pulse Rectifier Recipe to ListBox.vi"("Right AmpMins"=w334, "Left AmpMins"=w337, "Right Amps"=w335, "Left Amps"=w338, "error in (no error)"=w333, "Number Steps"=w336, "ListBox"=w330) -> ("error out"=w340:errorcluster)  [unwired: 4 in]
            n162 = local write "Reverse Current Multiplier"(w327) -> ()
            n163 = Number To Decimal String(number=w336) -> (decimal integer string=w343:string)  [unwired: 1 in]
            n164 = Bundle By Name(cluster=w341, "Data Type"=Data_Types."I32", "Name"="HMI_Rect1_2_NumSteps", "Value"=w343) -> (w347:T1)
            n165 = Flatten To String(anything=w347) -> (data string=w346:string)  [unwired: 3 in, 2 out]
            n166 = call <vilib>:"Send Local Message.vi"("message queue in"=w342, "message name"="Write_Tag", "message value"=w346, "error in"=w340) -> ("message queue out"=w345:T5, "error out"=w339:errorcluster)  [unwired: 9 in, 1 out]
            n167 = call <vilib>:"Send Local Message.vi"("message queue in"=w345, "message name"="UpdatePlatingMinutes", "message value"=w343, "error in"=w339) -> ("error out"=w329:errorcluster)  [unwired: 9 in, 2 out]
          }
          frame True {
          }
        }
      }
      frame "EZRecipe" {
        w363 = T7 7 items=["User Home"=0, "User Desktop"=1, "User Documents"=2, "User Application Data"=3, "User Preferences"=4, "User Temporary"=5, "Public Documents"=6, "Public Application Data"=7, "Public Preferences"=8, "Public Cache"=13, "System Core Libraries"=9, "System Installed Libraries"=10, "Application Files"=11, "Boot Volume Root"=12] ("system directory type")
        n168 = call <vilib>:"Get System Directory.vi"("system directory type"=w363) -> ("system directory"=w362:path)  [unwired: 10 in]
        n169 = local read "Loaded Recipe"() -> (w359:string)
        n170 = Build Path(base path=w362, name or relative path="TDK\\CDL0100") -> (appended path=w360:path)
        n171 = Build Path(base path=w360, name or relative path=w359) -> (appended path=w358:path)
        n172 = call "CDL0100 Recipe Creator v1.1.vi"("Previous Recipe Path"=w358) -> ("New Recipe Path"=w356:path, "canceled?"=w357:bool)  [unwired: 1 out]
        n173 = case shown="False" w357 {
          tunnel: w356 -> [w381 _]
          tunnel: w355 -> [w380 w387]
          tunnel: w354 -> [w370 _]
          tunnel: w353 -> [w366 _]
          tunnel: [w364 w387] -> w352
          frame False {
            n174 = control-ref of="Rectifer Settings"() -> (w368:refnum<vi>)
            n175 = call "Read Rectifier Recipe.vi"("selected path"=w381, "error in"=w380) -> ("Left Amps"=w386:dbl[], "Left AmpMins"=w385:dbl[], "Num Steps"=w369:i32, "name"=w367:string, "Right Amps"=w384:dbl[], "Right AmpMins"=w383:dbl[], "error out"=w382:errorcluster)  [unwired: 5 in, 2 out]
            n176 = call "Write Pulse Rectifier Recipe to ListBox.vi"("Right AmpMins"=w383, "Left AmpMins"=w385, "Right Amps"=w384, "Left Amps"=w386, "error in (no error)"=w382, "Number Steps"=w369, "ListBox"=w368) -> ("error out"=w365:errorcluster)  [unwired: 4 in]
            n177 = local write "Loaded Recipe"(w367) -> ()
            n178 = Number To Decimal String(number=w369) -> (decimal integer string=w372:string)  [unwired: 1 in]
            n179 = Bundle By Name(cluster=w370, "Data Type"=Data_Types."I32", "Name"="HMI_Rect1_2_NumSteps", "Value"=w372) -> (w376:T1)
            n180 = Flatten To String(anything=w376) -> (data string=w375:string)  [unwired: 3 in, 2 out]
            n181 = call <vilib>:"Send Local Message.vi"("message queue in"=w366, "message name"="Write_Tag", "message value"=w375, "error in"=w365) -> ("message queue out"=w374:T5, "error out"=w371:errorcluster)  [unwired: 9 in, 1 out]
            n182 = call <vilib>:"Send Local Message.vi"("message queue in"=w374, "message name"="UpdatePlatingMinutes", "message value"=w372, "error in"=w371) -> ("error out"=w364:errorcluster)  [unwired: 9 in, 2 out]
          }
          frame True {
          }
        }
      }
    }
  }
  n183 = while "Message Generator - User Interface Event Handler" {
    tunnel: w20 -> [w389]
    tunnel: w1 -> [w388]
    stop <- w390 stop-if-true
    w391 = 200  # Event Structure Timeout (ms)
    n184 = event shown="[24] \"EZ Recipe Button\": Value Change" {
      selector: _ -> [_ _ _ _ _ _ _ _ _ _ _ _ _ _ _ _ _ _ _ _ _ _ _ _ _ _ _ _ _ _ _ _ _ _ _ _ _ _ _ _ _ _ _]
      dyn-events: _ -> [_ _ _ _ _ _ _ _ _ _ _ _ _ _ _ _ _ _ _ _ _ _ _ _ _ _ _ _ _ _ _ _ _ _ _ _ _ _ _ _ _ _ _]
      timeout: w391 -> [_ _ _ _ _ _ _ _ _ _ _ _ _ _ _ _ _ _ _ _ _ _ _ _ _ _ _ _ _ _ _ _ _ _ _ _ _ _ _ _ _ _ _]
      tunnel: [w392 w402 _ TRUE ("Discard?") TRUE ("Discard?") TRUE ("Discard?") TRUE ("Discard?") TRUE ("Discard?") TRUE ("Discard?") TRUE ("Discard?") TRUE ("Discard?") TRUE ("Discard?") TRUE ("Discard?") TRUE ("Discard?") TRUE ("Discard?") TRUE ("Discard?") TRUE ("Discard?") TRUE ("Discard?") TRUE ("Discard?") TRUE ("Discard?") TRUE ("Discard?") FALSE ("Discard?") FALSE ("Discard?") FALSE ("Discard?") _ FALSE ("Discard?") FALSE ("Discard?") FALSE ("Discard?") FALSE ("Discard?") FALSE ("Discard?") FALSE ("Discard?") FALSE ("Discard?") FALSE ("Discard?") FALSE ("Discard?") FALSE ("Discard?") FALSE ("Discard?") _ _ _ _ FALSE ("Discard?") _ _] -> w390
      tunnel: w389 -> [w393 w400 _ w408 w413 w419 w424 w429 w434 w439 w444 w448 w453 w458 w463 w468 w473 w478 w483 w488 w493 w500 w504 w509 w513 w526 w537 w548 w559 w563 w577 w597 w607 w617 w627 w639 w641 w643 w648 w653 w659 w682 _]
      tunnel: w388 -> [_ _ _ _ _ _ _ _ _ _ _ _ _ _ _ _ _ _ _ _ _ _ _ _ _ w523 w534 w545 w556 w562 w576 w596 w606 w616 w626 w638 _ _ _ _ w658 _ _]
      event Timeout {
        n185 = event-data() -> ()  [unwired: 2 out]
        n186 = call "CheckForAutoLogout.vi"() -> ("Boolean"=w394:bool)  [unwired: 11 in]
        n187 = case shown="True" w394 {
          tunnel: [FALSE ("Discard?") TRUE ("Discard?")] -> w392
          tunnel: w393 -> [_ w396]
          frame False {
          }
          frame True {
            n188 = call <userlib>:"HNE Page Manager (Set).vi"("Next Page"="Home") -> ()  [unwired: 4 in, 1 out]
            n189 = call <vilib>:"Send Local Message.vi"("message queue in"=w396, "message name"="Exit") -> ()  [unwired: 11 in, 3 out]
          }
        }
      }
      event Panel Close? {
        w402 = TRUE ("Discard?")
        # "Intercepts the upper right close panel\noperation to allow a smooth shutdown\nas opposed to immediately killing the app."
        n190 = event-data() -> ()  [unwired: 2 out]
        n191 = call <vilib>:"Send Local Message.vi"("message queue in"=w400, "message name"="Exit") -> ()  [unwired: 11 in, 3 out]
        n192 = event-data("Discard?"=w402) -> ()  [unwired: 1 in, 1 out]
      }
      event Mouse Down? {
        n193 = event-data() -> ("Button"=w406:u16, "Mods"=w405:cluster{"Double Click":bool, "Menu Key":bool}, "PlatMods"=w404:T8)  [unwired: 6 out]
        n194 = Get Date/Time In Seconds() -> (seconds since 1Jan1904=w403:timestamp)
        n195 = shared-variable ".\\Local Variables.lvlib\\LastLogonTime"(w403) -> ()  [unwired: 1 in, 1 out]
        n196 = event-data("Button"=w406, "Mods"=w405, "PlatMods"=w404, "Discard?"=FALSE) -> ()  [unwired: 1 in, 1 out]
      }
      event "Machine": Value Change {
        # "Exit the application\n>> Stop this message generator loop"
        n197 = event-data() -> ()  [unwired: 2 out]
        n198 = call "Wait for Msg Complete.vi"("Queue in"=w408) -> ("Queue out"=w409:T5)  [unwired: 10 in]
        n199 = call <vilib>:"Send Local Message.vi"("message queue in"=w409, "message name"="Exit") -> ()  [unwired: 11 in, 3 out]
        n200 = call <userlib>:"HNE Page Manager (Set).vi"("Next Page"="Home") -> ()  [unwired: 4 in, 1 out]
      }
      event "Plater 2": Value Change {
        # "Exit the application\n>> Stop this message generator loop"
        n201 = event-data() -> ()  [unwired: 2 out]
        n202 = call "Wait for Msg Complete.vi"("Queue in"=w413) -> ("Queue out"=w414:T5)  [unwired: 10 in]
        n203 = call <userlib>:"HNE Page Manager (Set).vi"("Next Page"="Plater2") -> ()  [unwired: 4 in, 1 out]
        n204 = call <vilib>:"Send Local Message.vi"("message queue in"=w414, "message name"="Exit") -> ()  [unwired: 11 in, 3 out]
      }
      event "Plater 3": Value Change {
        # "Exit the application\n>> Stop this message generator loop"
        n205 = event-data() -> ()  [unwired: 2 out]
        n206 = call "Wait for Msg Complete.vi"("Queue in"=w419) -> ("Queue out"=w418:T5)  [unwired: 10 in]
        n207 = call <vilib>:"Send Local Message.vi"("message queue in"=w418, "message name"="Exit") -> ()  [unwired: 11 in, 3 out]
        n208 = call <userlib>:"HNE Page Manager (Set).vi"("Next Page"="Plater3") -> ()  [unwired: 4 in, 1 out]
      }
      event "Plater 4": Value Change {
        # "Exit the application\n>> Stop this message generator loop"
        n209 = event-data() -> ()  [unwired: 2 out]
        n210 = call "Wait for Msg Complete.vi"("Queue in"=w424) -> ("Queue out"=w423:T5)  [unwired: 10 in]
        n211 = call <vilib>:"Send Local Message.vi"("message queue in"=w423, "message name"="Exit") -> ()  [unwired: 11 in, 3 out]
        n212 = call <userlib>:"HNE Page Manager (Set).vi"("Next Page"="Plater4") -> ()  [unwired: 4 in, 1 out]
      }
      event "Plater 5": Value Change {
        # "Exit the application\n>> Stop this message generator loop"
        n213 = event-data() -> ()  [unwired: 2 out]
        n214 = call "Wait for Msg Complete.vi"("Queue in"=w429) -> ("Queue out"=w428:T5)  [unwired: 10 in]
        n215 = call <vilib>:"Send Local Message.vi"("message queue in"=w428, "message name"="Exit") -> ()  [unwired: 11 in, 3 out]
        n216 = call <userlib>:"HNE Page Manager (Set).vi"("Next Page"="Plater5") -> ()  [unwired: 4 in, 1 out]
      }
      event "Plater 6": Value Change {
        # "Exit the application\n>> Stop this message generator loop"
        n217 = event-data() -> ()  [unwired: 2 out]
        n218 = call "Wait for Msg Complete.vi"("Queue in"=w434) -> ("Queue out"=w433:T5)  [unwired: 10 in]
        n219 = call <vilib>:"Send Local Message.vi"("message queue in"=w433, "message name"="Exit") -> ()  [unwired: 11 in, 3 out]
        n220 = call <userlib>:"HNE Page Manager (Set).vi"("Next Page"="Plater6") -> ()  [unwired: 4 in, 1 out]
      }
      event "Rinse 2": Value Change {
        # "Exit the application\n>> Stop this message generator loop"
        n221 = event-data() -> ()  [unwired: 2 out]
        n222 = call "Wait for Msg Complete.vi"("Queue in"=w439) -> ("Queue out"=w438:T5)  [unwired: 10 in]
        n223 = call <vilib>:"Send Local Message.vi"("message queue in"=w438, "message name"="Exit") -> ()  [unwired: 11 in, 3 out]
        n224 = call <userlib>:"HNE Page Manager (Set).vi"("Next Page"="Rinse2") -> ()  [unwired: 4 in, 1 out]
      }
      event "Rinse 1": Value Change {
        # "Exit the application\n>> Stop this message generator loop"
        n225 = event-data() -> ()  [unwired: 2 out]
        n226 = call "Wait for Msg Complete.vi"("Queue in"=w444) -> ("Queue out"=w443:T5)  [unwired: 10 in]
        n227 = call <vilib>:"Send Local Message.vi"("message queue in"=w443, "message name"="Exit") -> ()  [unwired: 11 in, 3 out]
        n228 = call <userlib>:"HNE Page Manager (Set).vi"("Next Page"="Rinse1") -> ()  [unwired: 4 in, 1 out]
      }
      event "Rinse 3": Value Change {
        # "Exit the application\n>> Stop this message generator loop"
        n229 = event-data() -> ()  [unwired: 2 out]
        n230 = call "Wait for Msg Complete.vi"("Queue in"=w448) -> ("Queue out"=w449:T5)  [unwired: 10 in]
        n231 = call <vilib>:"Send Local Message.vi"("message queue in"=w449, "message name"="Exit") -> ()  [unwired: 11 in, 3 out]
        n232 = call <userlib>:"HNE Page Manager (Set).vi"("Next Page"="Rinse3") -> ()  [unwired: 4 in, 1 out]
      }
      event "Rinse 4": Value Change {
        # "Exit the application\n>> Stop this message generator loop"
        n233 = event-data() -> ()  [unwired: 2 out]
        n234 = call "Wait for Msg Complete.vi"("Queue in"=w453) -> ("Queue out"=w454:T5)  [unwired: 10 in]
        n235 = call <vilib>:"Send Local Message.vi"("message queue in"=w454, "message name"="Exit") -> ()  [unwired: 11 in, 3 out]
        n236 = call <userlib>:"HNE Page Manager (Set).vi"("Next Page"="Rinse4") -> ()  [unwired: 4 in, 1 out]
      }
      event "Dryer": Value Change {
        # "Exit the application\n>> Stop this message generator loop"
        n237 = event-data() -> ()  [unwired: 2 out]
        n238 = call "Wait for Msg Complete.vi"("Queue in"=w458) -> ("Queue out"=w459:T5)  [unwired: 10 in]
        n239 = call <vilib>:"Send Local Message.vi"("message queue in"=w459, "message name"="Exit") -> ()  [unwired: 11 in, 3 out]
        n240 = call <userlib>:"HNE Page Manager (Set).vi"("Next Page"="Dryer") -> ()  [unwired: 4 in, 1 out]
      }
      event "Predip": Value Change {
        # "Exit the application\n>> Stop this message generator loop"
        n241 = event-data() -> ()  [unwired: 2 out]
        n242 = call "Wait for Msg Complete.vi"("Queue in"=w463) -> ("Queue out"=w464:T5)  [unwired: 10 in]
        n243 = call <vilib>:"Send Local Message.vi"("message queue in"=w464, "message name"="Exit") -> ()  [unwired: 11 in, 3 out]
        n244 = call <userlib>:"HNE Page Manager (Set).vi"("Next Page"="Predip") -> ()  [unwired: 4 in, 1 out]
      }
      event "Cleaner": Value Change {
        # "Exit the application\n>> Stop this message generator loop"
        n245 = event-data() -> ()  [unwired: 2 out]
        n246 = call "Wait for Msg Complete.vi"("Queue in"=w468) -> ("Queue out"=w469:T5)  [unwired: 10 in]
        n247 = call <vilib>:"Send Local Message.vi"("message queue in"=w469, "message name"="Exit") -> ()  [unwired: 11 in, 3 out]
        n248 = call <userlib>:"HNE Page Manager (Set).vi"("Next Page"="Clean") -> ()  [unwired: 4 in, 1 out]
      }
      event "Etch": Value Change {
        # "Exit the application\n>> Stop this message generator loop"
        n249 = event-data() -> ()  [unwired: 2 out]
        n250 = call "Wait for Msg Complete.vi"("Queue in"=w473) -> ("Queue out"=w474:T5)  [unwired: 10 in]
        n251 = call <vilib>:"Send Local Message.vi"("message queue in"=w474, "message name"="Exit") -> ()  [unwired: 11 in, 3 out]
        n252 = call <userlib>:"HNE Page Manager (Set).vi"("Next Page"="Etch") -> ()  [unwired: 4 in, 1 out]
      }
      event "Basement 1": Value Change {
        # "Exit the application\n>> Stop this message generator loop"
        n253 = event-data() -> ()  [unwired: 2 out]
        n254 = call "Wait for Msg Complete.vi"("Queue in"=w478) -> ("Queue out"=w479:T5)  [unwired: 10 in]
        n255 = call <vilib>:"Send Local Message.vi"("message queue in"=w479, "message name"="Exit") -> ()  [unwired: 11 in, 3 out]
        n256 = call <userlib>:"HNE Page Manager (Set).vi"("Next Page"="Basement1") -> ()  [unwired: 4 in, 1 out]
      }
      event "Basement 2": Value Change {
        # "Exit the application\n>> Stop this message generator loop"
        n257 = event-data() -> ()  [unwired: 2 out]
        n258 = call "Wait for Msg Complete.vi"("Queue in"=w483) -> ("Queue out"=w484:T5)  [unwired: 10 in]
        n259 = call <vilib>:"Send Local Message.vi"("message queue in"=w484, "message name"="Exit") -> ()  [unwired: 11 in, 3 out]
        n260 = call <userlib>:"HNE Page Manager (Set).vi"("Next Page"="Basement2") -> ()  [unwired: 4 in, 1 out]
      }
      event "Basement 3": Value Change {
        # "Exit the application\n>> Stop this message generator loop"
        n261 = event-data() -> ()  [unwired: 2 out]
        n262 = call "Wait for Msg Complete.vi"("Queue in"=w488) -> ("Queue out"=w489:T5)  [unwired: 10 in]
        n263 = call <vilib>:"Send Local Message.vi"("message queue in"=w489, "message name"="Exit") -> ()  [unwired: 11 in, 3 out]
        n264 = call <userlib>:"HNE Page Manager (Set).vi"("Next Page"="Basement3") -> ()  [unwired: 4 in, 1 out]
      }
      event "Basement 4": Value Change {
        # "Exit the application\n>> Stop this message generator loop"
        n265 = event-data() -> ()  [unwired: 2 out]
        n266 = call "Wait for Msg Complete.vi"("Queue in"=w493) -> ("Queue out"=w494:T5)  [unwired: 10 in]
        n267 = call <vilib>:"Send Local Message.vi"("message queue in"=w494, "message name"="Exit") -> ()  [unwired: 11 in, 3 out]
        n268 = call <userlib>:"HNE Page Manager (Set).vi"("Next Page"="Basement4") -> ()  [unwired: 4 in, 1 out]
      }
      event "Enable Plating Cell": Value Change {
        n269 = event-data() -> ("NewVal"=w501:bool)  [unwired: 1 out]
        n270 = call "Validate Plate Tank Enable.vi"("Valve No."=127, "Test Value"=w501, "Tag"="HMI_Tank1_Enable", "Queue in"=w500) -> ()  [unwired: 8 in]
      }
      event "Save This Recipe": Value Change {
        n271 = event-data() -> ("NewVal"=w503:bool)  [unwired: 1 out]
        n272 = case shown="True" w503 {
          tunnel: w504 -> [_ w507]
          frame False {
          }
          frame True {
            n273 = call <vilib>:"Send Local Message.vi"("message queue in"=w507, "message name"="Save_Recipe") -> ()  [unwired: 11 in, 3 out]
          }
        }
      }
      event "Load A Recipe": Value Change {
        n274 = event-data() -> ("NewVal"=w508:bool)  [unwired: 1 out]
        n275 = case shown="True" w508 {
          tunnel: w509 -> [_ w512]
          frame False {
          }
          frame True {
            n276 = call <vilib>:"Send Local Message.vi"("message queue in"=w512, "message name"="Load_A_Recipe") -> ()  [unwired: 11 in, 3 out]
          }
        }
      }
      event "EZ Recipe Button": Value Change {
        n277 = event-data() -> ("NewVal"=w514:bool)  [unwired: 6 out]
        n278 = case shown="True" w514 {
          tunnel: w513 -> [_ w515]
          frame False {
          }
          frame True {
            n279 = call <vilib>:"Send Local Message.vi"("message queue in"=w515, "message name"="EZRecipe") -> ()  [unwired: 11 in, 3 out]
          }
        }
      }
      event "Full Drain Plating Cell": Value Change {
        n280 = event-data() -> ("NewVal"=w525:bool)  [unwired: 1 out]
        n281 = Boolean To (0,1)(Boolean=w525) -> (0, 1=w524:i16)
        n282 = Number To Decimal String(number=w524) -> (decimal integer string=w520:string)  [unwired: 1 in]
        n283 = Bundle By Name(cluster=w523, "Data Type"=Data_Types."Boolean", "Name"="HMI_Tank1_Drain", "Value"=w520) -> (w519:T1)
        n284 = Flatten To String(anything=w519) -> (data string=w518:string)  [unwired: 3 in, 2 out]
        n285 = call <vilib>:"Send Local Message.vi"("message queue in"=w526, "message name"="Write_Tag", "message value"=w518) -> ()  [unwired: 10 in, 3 out]
      }
      event "Enable Eductor Motion": Value Change {
        n286 = event-data() -> ("NewVal"=w536:bool)  [unwired: 1 out]
        n287 = Boolean To (0,1)(Boolean=w536) -> (0, 1=w535:i16)
        n288 = Number To Decimal String(number=w535) -> (decimal integer string=w531:string)  [unwired: 1 in]
        n289 = Bundle By Name(cluster=w534, "Data Type"=Data_Types."Boolean", "Name"="HMI_Tank1_Eductor_Motors_Run", "Value"=w531) -> (w530:T1)
        n290 = Flatten To String(anything=w530) -> (data string=w529:string)  [unwired: 3 in, 2 out]
        n291 = call <vilib>:"Send Local Message.vi"("message queue in"=w537, "message name"="Write_Tag", "message value"=w529) -> ()  [unwired: 10 in, 3 out]
      }
      event "Enable Rack Motion": Value Change {
        n292 = event-data() -> ("NewVal"=w547:bool)  [unwired: 1 out]
        n293 = Boolean To (0,1)(Boolean=w547) -> (0, 1=w546:i16)
        n294 = Number To Decimal String(number=w546) -> (decimal integer string=w542:string)  [unwired: 1 in]
        n295 = Bundle By Name(cluster=w545, "Data Type"=Data_Types."Boolean", "Name"="HMI_Tank1_Rack_Motor_Run", "Value"=w542) -> (w541:T1)
        n296 = Flatten To String(anything=w541) -> (data string=w540:string)  [unwired: 3 in, 2 out]
        n297 = call <vilib>:"Send Local Message.vi"("message queue in"=w548, "message name"="Write_Tag", "message value"=w540) -> ()  [unwired: 10 in, 3 out]
      }
      event "Enable Suck Pump": Value Change {
        n298 = event-data() -> ("NewVal"=w558:bool)  [unwired: 1 out]
        n299 = Boolean To (0,1)(Boolean=w558) -> (0, 1=w557:i16)
        n300 = Number To Decimal String(number=w557) -> (decimal integer string=w553:string)  [unwired: 1 in]
        n301 = Bundle By Name(cluster=w556, "Data Type"=Data_Types."Boolean", "Name"="HMI_Tnk1_Enable_SuckPump", "Value"=w553) -> (w552:T1)
        n302 = Flatten To String(anything=w552) -> (data string=w551:string)  [unwired: 3 in, 2 out]
        n303 = call <vilib>:"Send Local Message.vi"("message queue in"=w559, "message name"="Write_Tag", "message value"=w551) -> ()  [unwired: 10 in, 3 out]
      }
      event "Start Cycle": Value Change {
        n304 = event-data() -> ("NewVal"=w561:bool)  [unwired: 1 out]
        n305 = case shown="True" w561 {
          tunnel: w563 -> [_ w574]
          tunnel: w561 -> [_ w573]
          tunnel: w562 -> [_ w571]
          frame False {
          }
          frame True {
            n306 = Boolean To (0,1)(Boolean=w573) -> (0, 1=w572:i16)
            n307 = Number To Decimal String(number=w572) -> (decimal integer string=w568:string)  [unwired: 1 in]
            n308 = Bundle By Name(cluster=w571, "Data Type"=Data_Types."Boolean", "Name"="HMI_Rect1_2_Cycle", "Value"=w568) -> (w567:T1)
            n309 = Flatten To String(anything=w567) -> (data string=w566:string)  [unwired: 3 in, 2 out]
            n310 = call <vilib>:"Send Local Message.vi"("message queue in"=w574, "message name"="Write_Tag", "message value"=w566) -> ()  [unwired: 10 in, 3 out]
          }
        }
      }
      event "Cancel Cycle": Value Change {
        n311 = event-data() -> ("NewVal"=w575:bool)  [unwired: 1 out]
        n312 = case shown="True" w575 {
          tunnel: w577 -> [_ w588]
          tunnel: w575 -> [_ w587]
          tunnel: w576 -> [_ w585]
          frame False {
          }
          frame True {
            n313 = Boolean To (0,1)(Boolean=w587) -> (0, 1=w586:i16)
            n314 = Number To Decimal String(number=w586) -> (decimal integer string=w582:string)  [unwired: 1 in]
            n315 = Bundle By Name(cluster=w585, "Data Type"=Data_Types."Boolean", "Name"="HMI_Rect1_2_CycleStop", "Value"=w582) -> (w581:T1)
            n316 = Flatten To String(anything=w581) -> (data string=w580:string)  [unwired: 3 in, 2 out]
            n317 = call <vilib>:"Send Local Message.vi"("message queue in"=w588, "message name"="Write_Tag", "message value"=w580) -> ()  [unwired: 10 in, 3 out]
          }
        }
      }
      event "Eductor RPM": Value Change {
        n318 = event-data() -> ("NewVal"=w590:dbl)  [unwired: 1 out]
        n319 = Number To Fractional String(number=w590) -> (F-format string=w589:string)  [unwired: 3 in]
        n320 = Bundle By Name(cluster=w596, "Data Type"=Data_Types."Double", "Name"="HMI_Tnk1_Eductor_RPM", "Value"=w589) -> (w593:T1)
        n321 = Flatten To String(anything=w593) -> (data string=w592:string)  [unwired: 3 in, 2 out]
        n322 = call <vilib>:"Send Local Message.vi"("message queue in"=w597, "message name"="Write_Tag", "message value"=w592) -> ()  [unwired: 10 in, 3 out]
      }
      event "Rack RPM": Value Change {
        n323 = event-data() -> ("NewVal"=w600:dbl)  [unwired: 1 out]
        n324 = Number To Fractional String(number=w600) -> (F-format string=w599:string)  [unwired: 3 in]
        n325 = Bundle By Name(cluster=w606, "Data Type"=Data_Types."Double", "Name"="HMI_Tnk1_Rack_RPM", "Value"=w599) -> (w603:T1)
        n326 = Flatten To String(anything=w603) -> (data string=w602:string)  [unwired: 3 in, 2 out]
        n327 = call <vilib>:"Send Local Message.vi"("message queue in"=w607, "message name"="Write_Tag", "message value"=w602) -> ()  [unwired: 10 in, 3 out]
      }
      event "Total Inflow (L/min)": Value Change {
        n328 = event-data() -> ("NewVal"=w610:dbl)  [unwired: 1 out]
        n329 = Number To Fractional String(number=w610) -> (F-format string=w609:string)  [unwired: 3 in]
        n330 = Bundle By Name(cluster=w616, "Data Type"=Data_Types."Double", "Name"="HMI_TNK1_Flow_Setpoint", "Value"=w609) -> (w613:T1)
        n331 = Flatten To String(anything=w613) -> (data string=w612:string)  [unwired: 3 in, 2 out]
        n332 = call <vilib>:"Send Local Message.vi"("message queue in"=w617, "message name"="Write_Tag", "message value"=w612) -> ()  [unwired: 10 in, 3 out]
      }
      event "Supply Pressure (kPa)": Value Change {
        n333 = event-data() -> ("NewVal"=w620:dbl)  [unwired: 1 out]
        n334 = Number To Fractional String(number=w620) -> (F-format string=w619:string)  [unwired: 3 in]
        n335 = Bundle By Name(cluster=w626, "Data Type"=Data_Types."Double", "Name"="HMI_BAS_TNK1_P_Setpoint", "Value"=w619) -> (w623:T1)
        n336 = Flatten To String(anything=w623) -> (data string=w622:string)  [unwired: 3 in, 2 out]
        n337 = call <vilib>:"Send Local Message.vi"("message queue in"=w627, "message name"="Write_Tag", "message value"=w622) -> ()  [unwired: 10 in, 3 out]
      }
      event "Suck Pump fraction of inflow": Value Change {
        n338 = event-data() -> ("NewVal"=w630:dbl)  [unwired: 1 out]
        n339 = Divide(x=w630, y=100.0) -> (x/y=w629:dbl)
        n340 = Number To Fractional String(number=w629) -> (F-format string=w632:string)  [unwired: 3 in]
        n341 = Bundle By Name(cluster=w638, "Data Type"=Data_Types."Double", "Name"="HMI_TNK1_SuckPmpFrac_Setpoint", "Value"=w632) -> (w635:T1)
        n342 = Flatten To String(anything=w635) -> (data string=w634:string)  [unwired: 3 in, 2 out]
        n343 = call <vilib>:"Send Local Message.vi"("message queue in"=w639, "message name"="Write_Tag", "message value"=w634) -> ()  [unwired: 10 in, 3 out]
      }
      event Menu Selection (User) {
        # "Add run-time menu items to the message\nqueue. The message handler case names must match the menu ItemTag names."
        n344 = event-data() -> ("ItemTag"=w642:string)  [unwired: 1 out]
        n345 = call <vilib>:"Send Local Message.vi"("message queue in"=w641, "message name"=w642) -> ()  [unwired: 11 in, 3 out]
      }
      event "Cell T Last Hr": Value Change {
        n346 = event-data() -> ("NewVal"=w644:bool)  [unwired: 3 out]
        n347 = case shown="True" w644 {
          tunnel: w643 -> [_ w647]
          frame False {
          }
          frame True {
            n348 = call <vilib>:"Send Local Message.vi"("message queue in"=w647, "message name"="DisplayLastHr", "message value"="TNK1_Temperature") -> ()  [unwired: 10 in, 3 out]
          }
        }
      }
      event "BasT1_Level Last Hr": Value Change {
        n349 = event-data() -> ("NewVal"=w649:bool)  [unwired: 3 out]
        n350 = case shown="True" w649 {
          tunnel: w648 -> [_ w652]
          frame False {
          }
          frame True {
            n351 = call <vilib>:"Send Local Message.vi"("message queue in"=w652, "message name"="DisplayLastHr", "message value"="BAS_Proc1_Tank_Level") -> ()  [unwired: 10 in, 3 out]
          }
        }
      }
      event "BasT1_P Last Hr": Value Change {
        n352 = event-data() -> ("NewVal"=w654:bool)  [unwired: 3 out]
        n353 = case shown="True" w654 {
          tunnel: w653 -> [_ w657]
          frame False {
          }
          frame True {
            n354 = call <vilib>:"Send Local Message.vi"("message queue in"=w657, "message name"="DisplayLastHr", "message value"="TNK12_MainPressure") -> ()  [unwired: 10 in, 3 out]
          }
        }
      }
      event "Rectifer Settings": Mouse Down {
        n355 = event-data() -> ("CtlRef"=w665:refnum<vi>, "Coords"=w664:T9, "Button"=w666:u16)  [unwired: 6 out]
        n356 = call "Handle Rectifer Step Selection.vi"("Coords"=w664, "Button"=w666, "MulticolumnListbox in"=w665) -> ("Row"=w660:i32)  [unwired: 8 in]
        n357 = Greater?(x=w660, y=0) -> (0:w661:bool)
        n358 = case shown="True" w661 {
          tunnel: w660 -> [_ w673]
          tunnel: w659 -> [_ w676]
          tunnel: w658 -> [_ w674]
          frame False {
          }
          frame True {
            n359 = Number To Decimal String(number=w673) -> (decimal integer string=w667:string)  [unwired: 1 in]
            n360 = Bundle By Name(cluster=w674, "Data Type"=Data_Types."I32", "Name"="HMI_Rect1_2_NumSteps", "Value"=w667) -> (w671:T1)
            n361 = Flatten To String(anything=w671) -> (data string=w670:string)  [unwired: 3 in, 2 out]
            n362 = call <vilib>:"Send Local Message.vi"("message queue in"=w676, "message name"="Write_Tag", "message value"=w670) -> ("message queue out"=w669:T5)  [unwired: 10 in, 2 out]
            n363 = call <vilib>:"Send Local Message.vi"("message queue in"=w669, "message name"="UpdatePlatingMinutes", "message value"=w667) -> ()  [unwired: 10 in, 3 out]
          }
        }
      }
      event "Rectifer Settings": Edit Cell {
        n364 = event-data() -> ("CtlRef"=w687:refnum<vi>, "String"=w685:string, "Coords"=w686:T10)  [unwired: 4 out]
        n365 = call "Data Check Rectifier Settings.vi"("String"=w685, "Coords"=w686, "MulticolumnListbox in"=w687) -> ("error out"=w678:errorcluster)  [unwired: 7 in, 1 out]
        n366 = shared-variable-read(refnum<k21> "ni.var.psp://z004551/CDL0100 ReadWriteTags/HMI_Rect1_2_NumSteps" ("shared variable refnum in"), 0) -> (w680:i32)  [unwired: 1 in, 3 out]
        n367 = Number To Decimal String(number=w680) -> (decimal integer string=w679:string)  [unwired: 1 in]
        n368 = call <vilib>:"Send Local Message.vi"("message queue in"=w682, "message name"="UpdatePlatingMinutes", "message value"=w679, "error in"=w678) -> ()  [unwired: 9 in, 3 out]
      }
      event "MO": Value Change {
        n369 = event-data() -> ("NewVal"=w688:string)  [unwired: 6 out]
        n370 = shared-variable ".\\Local Variables.lvlib\\PT1_MO"(w688) -> ()  [unwired: 1 in, 1 out]
      }
    }
  }
  n371 = call-poly <vilib>:"Get Connection Reference.vi"("error in"=w8, "connection info in"=w9) -> ("error out"=w12:errorcluster, "connection ID out"=w11:refnum<k5>)  [unwired: 8 out]
  n372 = TCP Close Connection(connection ID=w11, error in (no error)=w12) -> (error out=w14:errorcluster)  [unwired: 2 out]
  n373 = call <vilib>:"Error to Warning.vi"("1st Error to Convert"=w13, "error in"=w14) -> ("warning out"=w10:errorcluster)  [unwired: 3 in, 10 out]
  n374 = call <vilib>:"Simple Error Handler.vi"("error in (no error)"=w10) -> ()  [unwired: 4 in, 5 out]
